vi "TestContinuity.vi"(4 "Voltage Limit DxBoot0":dbl, 5 "Voltage Limit DxSupply":dbl, 6 "Current Level DxBoot0":dbl, 7 "Current Level DxSupply":dbl, 8 "error in (no error)":errorcluster, 9 "DxBoot0":string="0", 10 "DxSupply":string="0", 11 "IVI Refnum in":refnum<k15>) -> (0 "error out":errorcluster, 1 "Volt Average DxSupply":dbl format="%0.2f", 2 "Volt Average DxBoot0":dbl format="%0.2f")   [LabVIEW 2018]
uses:
  <instrlib>/niDCPower/nidcpower.llb/niDCPower Measurement Type.ctl
  <vilib>/Analysis/baseanly.llb/Mean (DBL).vi
  <vilib>/Analysis/NI_AALBase.lvlib
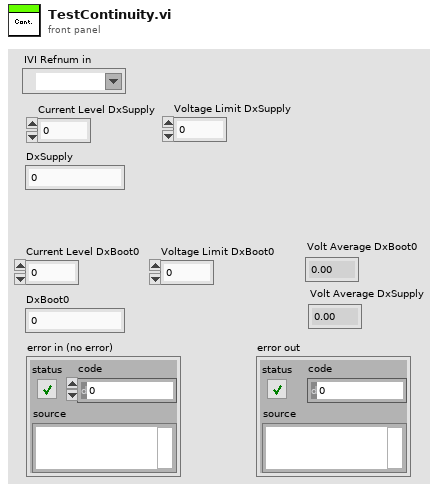
[diagram p1: front panel]
types:
  T1 = typedef "niDCPower Measurement Type.ctl" = i32
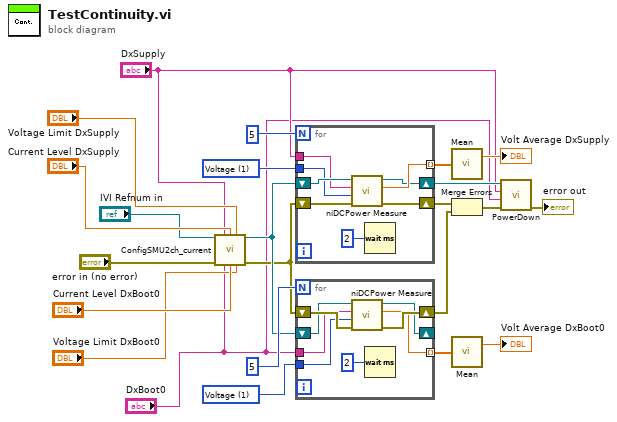
[diagram p0: block diagram]
diagram:
  w16 = T1 1 items=["Current", "Voltage"] ("measurement type")
  w20 = T1 1 items=["Current", "Voltage"] ("measurement type")
  n1 = call "ConfigSMU2ch_current.vi"("IVI Refnum in"="IVI Refnum in", "Channel DxSupply"="DxSupply", "Current Level DxSupply"="Current Level DxSupply", "Voltage Limit DxSupply"="Voltage Limit DxSupply", "error in (no error)"="error in (no error)", "Channel DxBoot0"="DxBoot0", "Current Level DxBoot0"="Current Level DxBoot0", "Voltage Limit DxBoot0"="Voltage Limit DxBoot0") -> ("IVI Refnum out"=w9:refnum<k15>, "error out"=w8:errorcluster)  [unwired: 6 in]
  n2 = for {
    N: 5 -> [_]
    tunnel: [w29] -> w18 mode=indexing
    shift-right: [w30] -> w5
    shift-left: w8 -> [w31]
    shift-right: [w28] -> w3
    shift-left: w9 -> [w27]
    tunnel: w16 -> [w26]
    tunnel: "DxSupply" -> [w25]
    n3 = call <instrlib>:"niDCPower Measure.vi"("error in (no error)"=w31, "measurement type"=w26, "channel name"=w25, "instrument handle"=w27) -> ("error out"=w30:errorcluster, "measurement"=w29:dbl, "instrument handle out"=w28:refnum<k15>)  [unwired: 5 in]
    n4 = Wait (ms)(milliseconds to wait=u32 2) -> ()  [unwired: 1 out]
  }
  n5 = for {
    N: 5 -> [_]
    tunnel: [w37] -> w22 mode=indexing
    shift-right: [w38] -> w4
    shift-left: w8 -> [w39]
    shift-right: [w36] -> _
    shift-left: w9 -> [w35]
    tunnel: w20 -> [w34]
    tunnel: "DxBoot0" -> [w33]
    n6 = call <instrlib>:"niDCPower Measure.vi"("error in (no error)"=w39, "measurement type"=w34, "channel name"=w33, "instrument handle"=w35) -> ("error out"=w38:errorcluster, "measurement"=w37:dbl, "instrument handle out"=w36:refnum<k15>)  [unwired: 5 in]
    n7 = Wait (ms)(milliseconds to wait=u32 2) -> ()  [unwired: 1 out]
  }
  n8 = call-poly <vilib>:"Mean.vi"("X"=w18) -> ("mean"=→"Volt Average DxSupply":dbl)  [unwired: 1 out]
  n9 = Merge Errors(w5, w4) -> (w14:errorcluster)
  n10 = call-poly <vilib>:"Mean.vi"("X"=w22) -> ("mean"=→"Volt Average DxBoot0":dbl)  [unwired: 1 out]
  n11 = call "PowerDown.vi"("error in (no error)"=w14, "DxBoot0"="DxBoot0", "DxSupply"="DxSupply", "SMU handle in"=w3) -> ("error out"=→"error out":errorcluster)  [unwired: 6 in, 1 out]
